vi "Do.vi"(8 "error in":errorcluster, 10 "Actor in":refnum<class "Actor.lvclass">, 11 "Enable Compressor MSG":refnum<class "Enable Compressor MSG.lvclass">) -> (0 "error out":errorcluster, 2 "Actor out":refnum<class "Actor.lvclass">)   [LabVIEW 2016, in "Enable Compressor MSG.lvclass"]
doc: "(<B>Filename</B>: Actor Framework.lvlib:Message.lvclass:Do.vi)\n\nDefines what a message does when it is received by an actor. Generally, a message instructs an actor to invoke one of its methods. By default, this method does nothing. A child class must override it to define behavior. Create a child class by using the Actor Framework Message Maker dialog box."
uses:
  Enable Compressor MSG.lvclass
  gController.lvclass
  <vilib>/rvi/interface/nirviReadWriteControl/nirviReadWriteControl.xnode
  FPGA Ref.ctl
  FPGA Bitfiles/NickIO.lvbitx
  <vilib>/rvi/errors/niLvFpgaMergeErrorWithErrorCode.vi
  <vilib>/rvi/errors/niLvFpgaAdjustHostInterfaceError.vi
  <vilib>/ActorFramework/Actor/Actor.lvclass
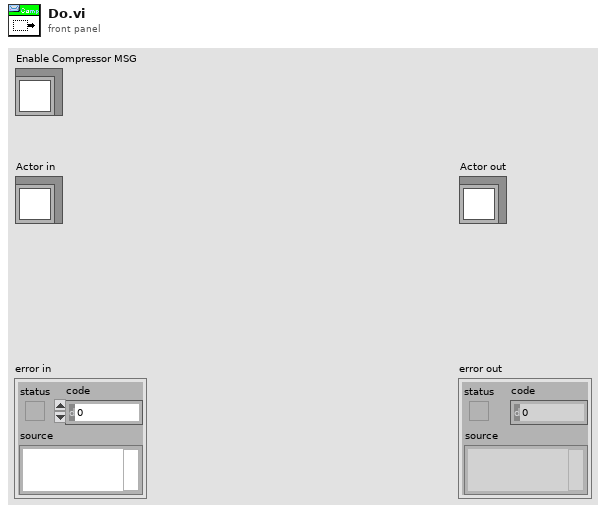
[diagram p1: front panel]
types:
  T1 = typedef "FPGA Ref.ctl" = refnum<k20>
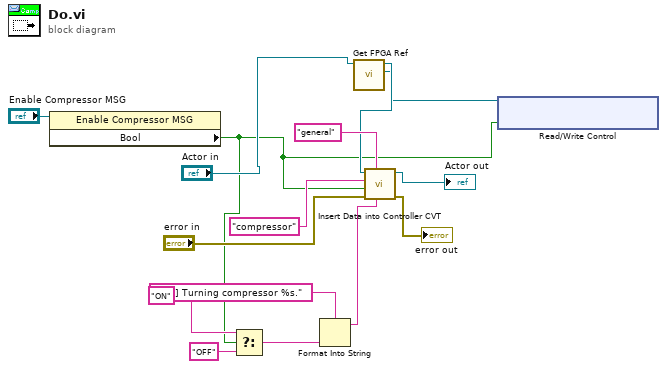
[diagram p0: block diagram]
diagram:
  n1 = property class="Enable Compressor MSG"(reference="Enable Compressor MSG") -> ("Bool"=w1:bool)  [unwired: 1 in, 2 out]
  n2 = Select(t="ON", s=w1, f="OFF") -> (s? t:f=w7:string)
  n3 = Format Into String(format string="[ctll] Turning compressor %s.", w7) -> (resulting string=w5:string)  [unwired: 2 in, 1 out]
  n4 = call "Get FPGA Ref.vi"("Actor In"="Actor in") -> ("FPGA Ref"=w2:T1, "Actor Out"=w3:refnum<class "Actor.lvclass">)  [unwired: 8 in, 1 out]
  n5 = call "Insert Data into Controller CVT.vi"("Update MSG"=w5, "Group"="general", "error in"="error in", "Data"=w1, "tag"="compressor", "Actor in"=w3) -> ("error out"=→"error out":errorcluster, "Actor Out"=→"Actor out":refnum<class "Actor.lvclass">)  [unwired: 4 in]
  n6 = xnode "Read/Write Control"("FPGA VI Reference In"=w2, "Compressor Enable"=w1) -> ()  [unwired: 1 in, 2 out]
